vi "SEND EMAILS.vi"(6 "Subject":string="PSC Item Reminder", 7 "USER EMAIL IN":string, 9 "SEND EMAIL":bool=TRUE, 10 "MESSAGE IN":string, 11 "connection reference in":T1) -> (3 "connection reference out":T1)   [LabVIEW 2019]
uses:
  <vilib>/addons/database/Connection.llb/Conn ObjectReference.ctl
  <vilib>/regexp/Match Regular Expression.xnode
  <vilib>/addons/database/NI_Database_API.lvlib
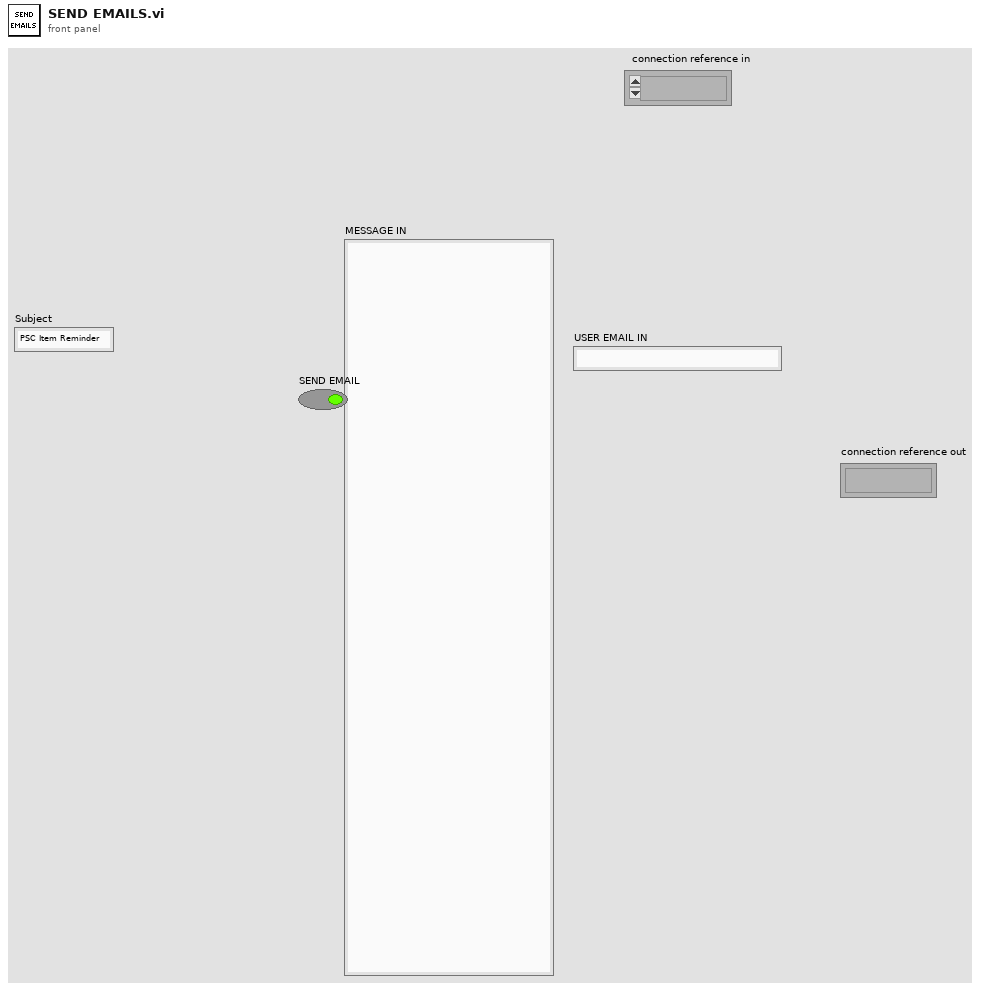
[diagram p1: front panel]
types:
  T1 = typedef "NI_Database_API.lvlib/Conn ObjectReference.ctl" = refnum<k1>
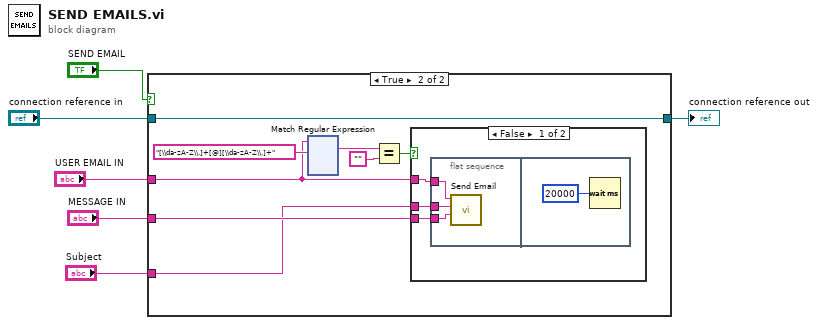
[diagram p0: block diagram]
diagram:
  n1 = case shown="True" "SEND EMAIL" {
    tunnel: "MESSAGE IN" -> [_ w14]
    tunnel: "USER EMAIL IN" -> [_ w11]
    tunnel: "connection reference in" -> [w7 w15]
    tunnel: [w7 w15] -> w2
    tunnel: "Subject" -> [_ w8]
    frame False {
    }
    frame True {
      n2 = xnode "Match Regular Expression"("input string"=w11, "regular expression"="[\\da-zA-Z\\.]+[@][\\da-zA-Z\\.]+" ("search string")) -> ("whole match"=w12:string)  [unwired: 4 in, 4 out]
      n3 = Equal?(x=w12, y="") -> (x = y?=w10:bool)
      n4 = case shown="False" w10 {
        tunnel: w11 -> [w132 _]
        tunnel: w8 -> [w131 _]
        tunnel: w14 -> [w130 _]
        frame False {
          n5 = flat-sequence {
            tunnel: w132 -> [w135]
            tunnel: w131 -> [w134]
            tunnel: w130 -> [w133]
            frame #0 {
              n6 = call "Send Email"("Message"=w133, "Subject"=w134, "Recipients"=w135) -> ()  [unwired: 8 in, 1 out]
            }
            frame #1 {
              n7 = Wait (ms)(milliseconds to wait=u32 20000) -> ()  [unwired: 1 out]
            }
          }
        }
        frame True {
        }
      }
    }
  }
  "connection reference out" <- w2
